vi "LINC Write Telemetry (Raw).vi"(8 "error in (no error)":errorcluster, 10 "raw packet":string, 11 "LINC session":refnum<class "LINC.lvclass">) -> (0 "error out":errorcluster, 3 "dup LINC session":refnum<class "LINC.lvclass">)   [LabVIEW 2018, in "STEPkgDriver_LINC.lvlib" / "LINC.lvclass"]
uses:
  LINC.lvclass
  STEPkgDriver_LINC.lvlib
  LINC Global Session Mode.ctl
  LINC Port Config.ctl
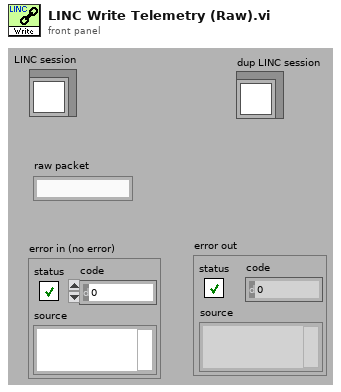
[diagram p1: front panel]
types:
  T1 = typedef "STEPkgDriver_LINC.lvlib/LINC Global Session Mode.ctl" = enum16{"INIT", "CLEAR", "ADD_SESSION", "SET_CONNECTION", "SET_LISTENER", "SET_REFERENCE", "GET_SESSION"}
  T2 = typedef "STEPkgDriver_LINC.lvlib/LINC Port Config.ctl" = enum16{"ALL", "CMD_ALL", "TLM_ALL", "TLM_BASIC"}
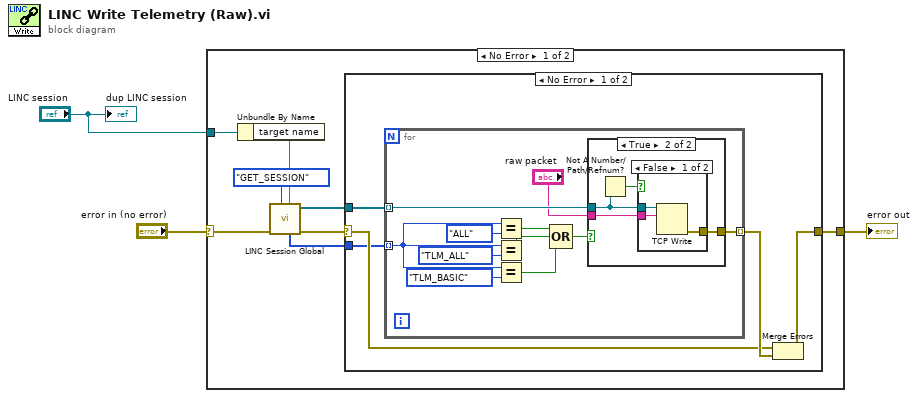
[diagram p0: block diagram]
diagram:
  n1 = case shown="No Error" "error in (no error)" {
    selector: "error in (no error)" -> [w4 w36]
    tunnel: [w11 w36] -> w3
    tunnel: "LINC session" -> [w10 _]
    frame No Error {
      n2 = Unbundle By Name(w10) -> ("target name"=w9:string)
      n3 = call "LINC Session Global.vi"("target name"=w9, "mode"=LINC_Global_Session_Mode."GET_SESSION", "error in (no error)"=w4) -> ("error out"=w6:errorcluster, "connections out"=w7:refnum<k5>[], "port config"=w5:T2[])  [unwired: 4 in, 2 out]
      n4 = case shown="No Error" w6 {
        selector: w6 -> [w13 w35]
        tunnel: w7 -> [w16 _]
        tunnel: [w14 w35] -> w11
        tunnel: w5 -> [w12 _]
        frame No Error {
          n5 = for {
            tunnel: w16 -> [w27] mode=indexing
            tunnel: [w26] -> w15 mode=indexing
            tunnel: w12 -> [w22] mode=indexing
            n6 = Equal?(x=w22, y=LINC_Port_Config."ALL") -> (x = y?=w21:bool)
            n7 = Equal?(x=w22, y=LINC_Port_Config."TLM_ALL") -> (x = y?=w20:bool)
            n8 = Equal?(x=w22, y=LINC_Port_Config."TLM_BASIC") -> (x = y?=w18:bool)
            n9 = Compound Arithmetic op=OR(w21, w20, w18) -> (w19:bool)
            n10 = case shown="True" w19 {
              tunnel: "raw packet" -> [_ w31]
              tunnel: w27 -> [_ w30]
              tunnel: [_ w29] -> w26
              frame False {
              }
              frame True {
                n11 = Not A Number/Path/Refnum?(number/path/refnum=w30) -> (NaN/Path/Refnum?=w28:bool)
                n12 = case shown="False" w28 {
                  tunnel: w31 -> [w34 _]
                  tunnel: w30 -> [w33 _]
                  tunnel: [w32 _] -> w29
                  frame False {
                    n13 = TCP Write(connection ID=w33, data in=w34) -> (error out=w32:errorcluster)  [unwired: 1 in, 3 out]
                  }
                  frame True {
                  }
                }
              }
            }
          }
          n14 = Merge Errors(w13, w15) -> (w14:errorcluster)
        }
        frame Error {
        }
      }
    }
    frame Error {
    }
  }
  "error out" <- w3
  "dup LINC session" <- "LINC session"
